vi "GDSError_Log.vi"(2 "cases":T1=enum."AddError", 5 "error in (no error)":errorcluster, 9 "DeleteWhenRead":bool) -> (16 "ErrorArray":errorcluster[](array[cluster]), 19 "error out":errorcluster)   [LabVIEW 2016]
uses:
  <resource>/Framework/Providers/Open_GDS/ClassProviders/Common/Error/private/GDSError_LogCases.ctl
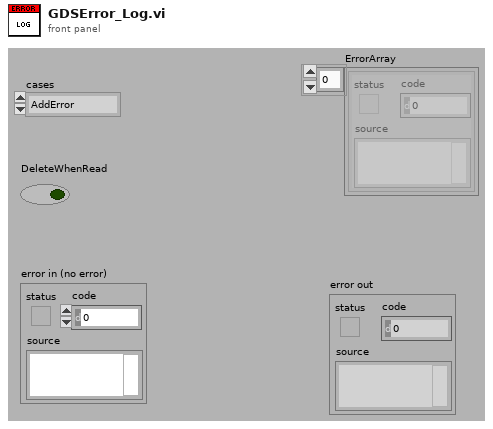
[diagram p1: front panel]
types:
  T1 = typedef "GDSError_LogCases.ctl" = enum16{"Init", "AddError", "ReadFirstError", "ReadLatestError", "ReadAllErrors", "ClearError", "ClearAllErrors"}
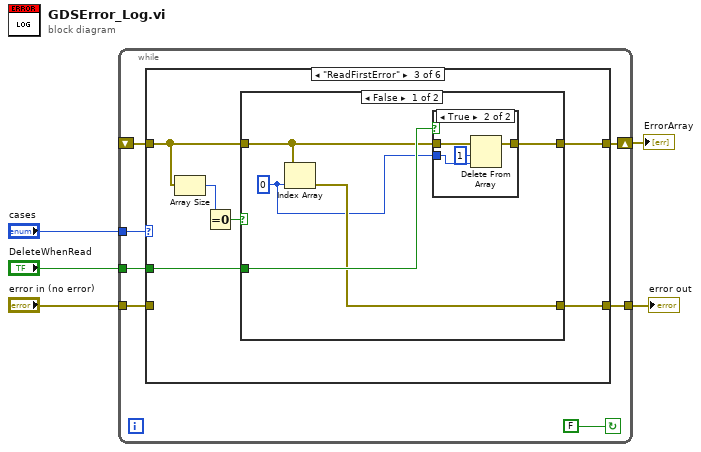
[diagram p0: block diagram]
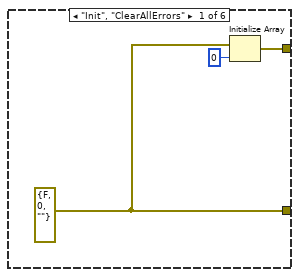
[diagram p2: hidden frame]
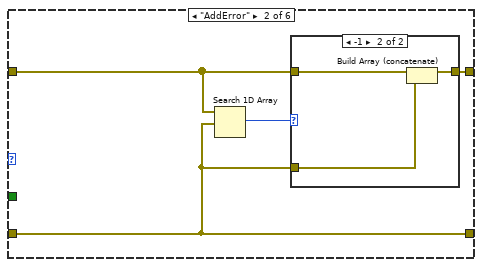
[diagram p3: hidden frame]
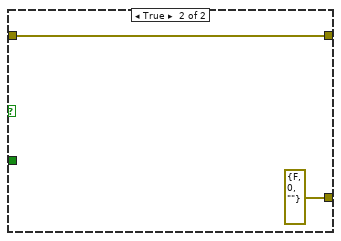
[diagram p6: hidden frame]
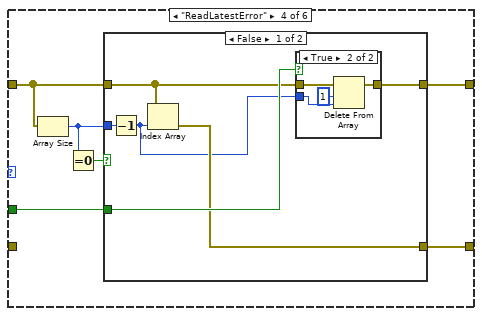
[diagram p7: hidden frame]
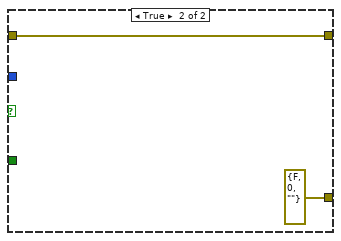
[diagram p9: hidden frame]
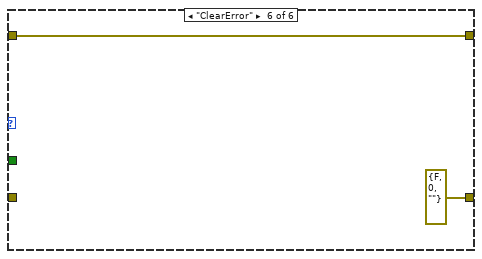
[diagram p11: hidden frame]
diagram:
  n1 = while {
    shift-right: [w10] -> w3
    shift-left: _ -> [w9]
    tunnel: "cases" -> [w11]
    tunnel: "error in (no error)" -> [w8]
    tunnel: [w7] -> w2
    tunnel: "DeleteWhenRead" -> [w6]
    stop <- FALSE continue-if-true
    n2 = case shown="\"ReadFirstError\"" w11 {
      tunnel: [w15 w19 w29 w47 w62 w64] -> w10
      tunnel: w9 -> [_ w16 w27 w45 w62 w64]
      tunnel: w8 -> [_ w17 _ _ w61 _]
      tunnel: [w13 w17 w26 w44 w61 errorcluster {"status"=FALSE, "code"=0, "source"=""} ("error in (no error)")] -> w7
      tunnel: w6 -> [_ _ w28 w46 _ _]
      frame "Init", "ClearAllErrors" {
        w13 = errorcluster {"status"=FALSE, "code"=0, "source"=""} ("error out")
        n3 = Initialize Array(w13, 0 ("dimension size")) -> (w15:errorcluster[])
      }
      frame "AddError" {
        n4 = Search 1D Array(1D array=w16, element=w17) -> (index of element=w18:i32)  [unwired: 1 in]
        n5 = case shown="-1" w18 {
          tunnel: [w20 w23] -> w19
          tunnel: w16 -> [w20 w22]
          tunnel: w17 -> [_ w21]
          frame 0.., Default {
            # "Error already\nadded"
          }
          frame -1 {
            n6 = Build Array (concatenate)(w22, w21) -> (w23:errorcluster[])
          }
        }
      }
      frame "ReadFirstError" {
        n7 = Array Size(array=w27) -> (size(s)=w24:i32)
        n8 = Equal To 0?(x=w24) -> (x = 0?=w25:bool)
        n9 = case shown="False" w25 {
          tunnel: [w34 w41] -> w29
          tunnel: w28 -> [w33 _]
          tunnel: w27 -> [w32 w41]
          tunnel: [w31 errorcluster {"status"=FALSE, "code"=0, "source"=""}] -> w26
          frame False {
            w30 = 0
            n10 = Index Array(array=w32, index=w30) -> (element=w31:errorcluster)
            n11 = case shown="True" w33 {
              tunnel: [w35 w37] -> w34
              tunnel: w32 -> [w35 w39]
              tunnel: w30 -> [_ w38]
              frame False {
              }
              frame True {
                n12 = Delete From Array(array=w39, length=1, index=w38) -> (array with subset deleted=w37:errorcluster[])  [unwired: 1 out]
              }
            }
          }
          frame True {
          }
        }
      }
      frame "ReadLatestError" {
        n13 = Array Size(array=w45) -> (size(s)=w43:i32)
        n14 = Equal To 0?(x=w43) -> (x = 0?=w42:bool)
        n15 = case shown="False" w42 {
          tunnel: [w53 w60] -> w47
          tunnel: w46 -> [w52 _]
          tunnel: w45 -> [w51 w60]
          tunnel: [w50 errorcluster {"status"=FALSE, "code"=0, "source"=""}] -> w44
          tunnel: w43 -> [w48 _]
          frame False {
            n16 = Decrement(x=w48) -> (x-1=w49:i32)
            n17 = Index Array(array=w51, index=w49) -> (element=w50:errorcluster)
            n18 = case shown="True" w52 {
              tunnel: [w54 w56] -> w53
              tunnel: w51 -> [w54 w58]
              tunnel: w49 -> [_ w57]
              frame False {
              }
              frame True {
                n19 = Delete From Array(array=w58, length=1, index=w57) -> (array with subset deleted=w56:errorcluster[])  [unwired: 1 out]
              }
            }
          }
          frame True {
          }
        }
      }
      frame "ReadAllErrors" {
      }
      frame "ClearError" {
      }
    }
  }
  "ErrorArray" <- w3
  "error out" <- w2
